vi "aoc-2025-d06-2.vi"() -> ()   [LabVIEW 2020]
panel:
  out "sum":i64
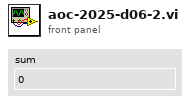
[diagram p1: front panel]
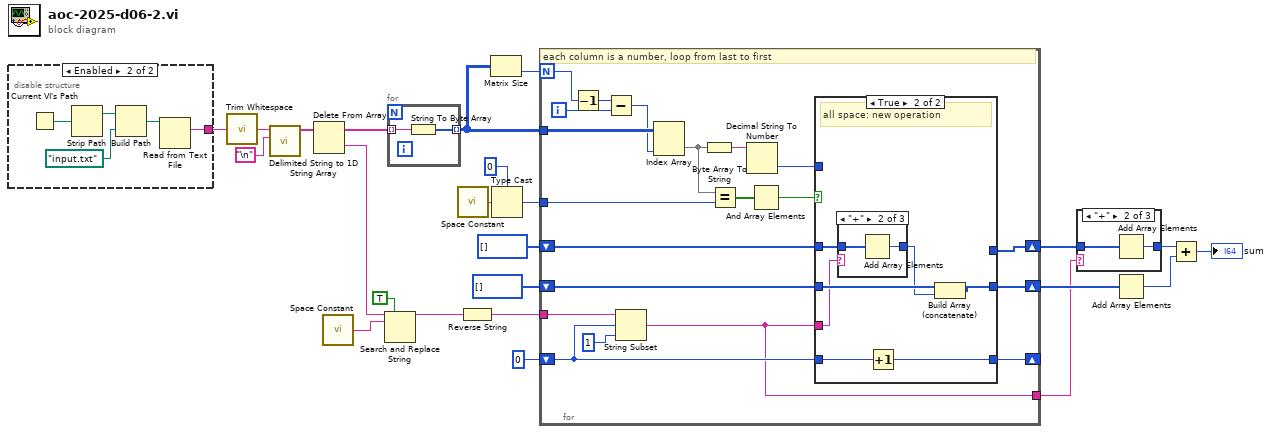
[diagram p0: block diagram]
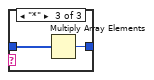
[diagram p3: hidden frame]
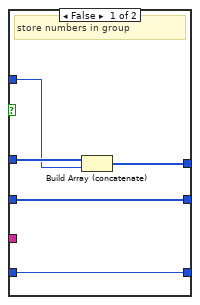
[diagram p4: hidden frame]
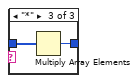
[diagram p6: hidden frame]
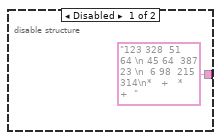
[diagram p7: hidden frame]
diagram:
  n1 = disable-structure shown="Enabled" {
    disable-tunnel: ["123 328  51 64 \n 45 64  387 23 \n  6 98  215 314\n*   +   *   +  " w26] -> w21
    frame Disabled {
    }
    frame Enabled {
      n2 = Current VI's Path() -> (path=w28:path)
      n3 = Strip Path(path=w28) -> (stripped path=w29:path)  [unwired: 1 out]
      n4 = Build Path(base path=w29, name or relative path=path "input.txt") -> (appended path=w30:path)
      n5 = Read from Text File(file (use dialog)=w30) -> (text=w26:string)  [unwired: 3 in, 3 out]
    }
  }
  n6 = call <vilib>:"Trim Whitespace.vi"("string"=w21) -> ("trimmed string"=w8:string)  [unwired: 1 in]
  n7 = call <vilib>:"Delimited String to 1D String Array.vi"("delimiter"="\n", "delimited string"=w8) -> ("string array"=w7:string[])  [unwired: 9 in]
  n8 = Delete From Array(array=w7) -> (deleted portion=w24:string, array with subset deleted=w20:string[])  [unwired: 2 in]
  n9 = call <vilib>:"Space Constant.vi"() -> ("String"=w17:string)
  n10 = Search and Replace String(replace all?=TRUE ("replace all? (F)"), input string=w24, search string=w17) -> (result string=w14:string)  [unwired: 5 in, 3 out]
  n11 = for {
    tunnel: w20 -> [w31] mode=indexing
    tunnel: [w32] -> w18 mode=indexing
    n12 = String To Byte Array(string=w31) -> (unsigned byte array=w32:u8[])
  }
  n13 = call <vilib>:"Space Constant.vi"() -> ("String"=w1:string)
  n14 = Reverse String(1:w14) -> (0:w11:string)
  n15 = Matrix Size(0:w18) -> (2:w19:i32)  [unwired: 1 out]
  n16 = Type Cast(type=u8 0, x=w1) -> (*(type *) &x=w15:u8)
  n17 = for {
    N: w19 -> [w51]
    tunnel: w18 -> [w49]
    tunnel: w15 -> [w48]
    tunnel: w11 -> [w46]
    shift-right: [w37] -> _
    shift-left: 0 -> [w38]
    shift-right: [w43] -> w5
    shift-left: i64[] [] -> [w35]
    shift-right: [w40] -> w9
    shift-left: i64[] [] -> [w39]
    tunnel: [w34] -> w6
    i -> [w52]
    # "each column is a number, loop from last to first"
    n18 = Decrement(x=w51) -> (x-1=w50:i32)
    n19 = Subtract(x=w50, y=w52) -> (x-y=w36:i32)
    n20 = String Subset(string=w46, offset (0)=w38, length (rest)=1 ("length (rest)")) -> (substring=w34:string)
    n21 = Index Array(array=w49, index (col)=w36) -> (element=w42:u8[])  [unwired: 1 in]
    n22 = Byte Array To String(unsigned byte array=w42) -> (string=w33:string)
    n23 = Equal?(x=w42, y=w48) -> (x = y?=w47:bool[])
    n24 = Decimal String To Number(string=w33) -> (number=w41:i32)  [unwired: 2 in, 1 out]
    n25 = And Array Elements(Boolean array=w47) -> (logical AND=w44:bool)
    n26 = case shown="True" w44 {
      tunnel: w34 -> [_ w60]
      tunnel: [w54 _] -> w43
      tunnel: w35 -> [w57 w59]
      tunnel: w41 -> [w55 _]
      tunnel: [w53 w64] -> w40
      tunnel: w39 -> [w53 w63]
      tunnel: w38 -> [w56 w62]
      tunnel: [w56 w61] -> w37
      frame False {
        # "store numbers in group"
        n27 = Build Array (concatenate)(w57, w55) -> (w54:i64[])
      }
      frame True {
        # "all space: new operation"
        n28 = case shown="\"+\"" w60 {
          tunnel: w59 -> [_ w66 w68]
          tunnel: [_ w65 w67] -> w58
          frame Default {
          }
          frame "+" {
            n29 = Add Array Elements(numeric array=w66) -> (sum=w65:i64)
          }
          frame "*" {
            n30 = Multiply Array Elements(1:w68) -> (0:w67:i64)
          }
        }
        n31 = Increment(x=w62) -> (x+1=w61:i32)
        n32 = Build Array (concatenate)(w63, w58) -> (w64:i64[])
      }
    }
  }
  n33 = case shown="\"+\"" w6 {
    tunnel: w5 -> [_ w70 w72]
    tunnel: [_ w69 w71] -> w3
    frame Default {
    }
    frame "+" {
      n34 = Add Array Elements(numeric array=w70) -> (sum=w69:i64)
    }
    frame "*" {
      n35 = Multiply Array Elements(1:w72) -> (0:w71:i64)
    }
  }
  n36 = Add Array Elements(numeric array=w9) -> (sum=w4:i64)
  n37 = Add(x=w3, y=w4) -> (x+y=→"sum":i64)
